vi "DAQ_build_waveform.vi"(0 "Résolution temporelle":dbl=1e-05 format="%#_6p", 1 "Décalage":dbl=0.0001 format="%#_6p", 2 "Largeur impulsion":dbl=0.25 format="%#_6p", 3 "Remise à 0":dbl=0.01 format="%#_6p", 4 "Pulse intensity":dbl=1.0 format="%#_6p") -> (5 "size(s)":i32, 6 "waveform":waveform(dbl), 7 "Digital waveform":digitalwaveform[](array[waveform]))   [LabVIEW 2015]
uses:
  <vilib>/Waveform/DWDTOps.llb/DWDT Analog to Digital.vi
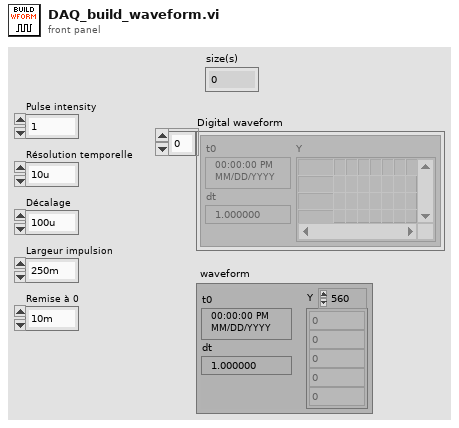
[diagram p1: front panel]
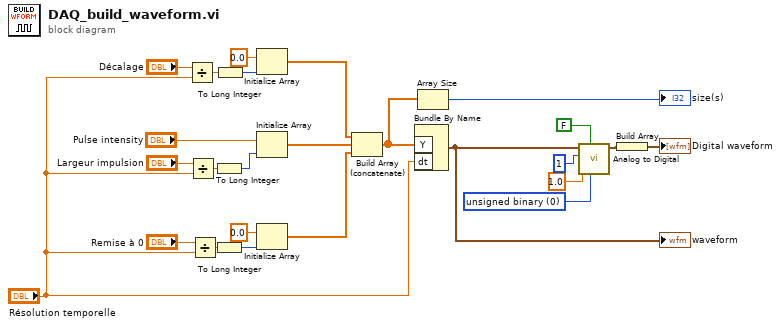
[diagram p0: block diagram]
diagram:
  w10 = u16 0 items=["unsigned binary", "offset binary", "2's complement"] ("data format (offset binary)")
  n1 = Divide(x="Décalage", y="Résolution temporelle") -> (x/y=w16:dbl)
  n2 = Divide(x="Largeur impulsion", y="Résolution temporelle") -> (x/y=w25:dbl)
  n3 = Divide(x="Remise à 0", y="Résolution temporelle") -> (x/y=w17:dbl)
  n4 = To Long Integer(number=w25) -> (32bit integer=w3:i32)
  n5 = To Long Integer(number=w17) -> (32bit integer=w2:i32)
  n6 = To Long Integer(number=w16) -> (32bit integer=w4:i32)
  n7 = Initialize Array(0.0 ("element"), w4) -> (w20:dbl[])
  n8 = Initialize Array("Pulse intensity", w3) -> (w19:dbl[])
  n9 = Initialize Array(0.0 ("element"), w2) -> (w18:dbl[])
  n10 = Build Array (concatenate)(w20, w19, w18) -> (w7:dbl[])
  n11 = Bundle By Name("Y"=w7, "dt"="Résolution temporelle") -> (w1:waveform(dbl))  [unwired: 1 in]
  "waveform" <- w1
  n12 = Array Size(array=w7) -> (size(s)=→"size(s)":i32)
  n13 = call-poly <vilib>:"Analog to Digital.vi"("data format (offset binary)"=w10, "compress digital (T)"=FALSE, "full-scale range (pk-pk)"=1.0, "resolution (16 bit)"=1, "analog waveform"=w1) -> ("digital waveform"=w12:digitalwaveform)  [unwired: 3 in, 3 out]
  n14 = Build Array(w12) -> (→"Digital waveform":digitalwaveform[])
